vi "Is_TestDataInSpec-1组数据相同规格.vi"(0 "相机量测结果":dbl[](array[numeric]), 1 "量测规格":T1 {"上限" format="%#.4g"; "下限" format="%#.4g"}) -> (3 "在规格内":bool, 4 "相机量测结果 out":dbl[](array[numeric]), 5 "数组":bool[](array[boolean]))   [LabVIEW 2014]
uses:
  Controls/TestThreshold.ctl
panel:
  # "~"
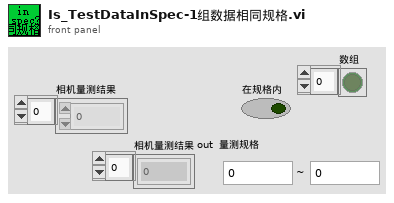
[diagram p1: front panel]
types:
  T1 = typedef "TestThreshold.ctl" = cluster{"下限":dbl, "上限":dbl}
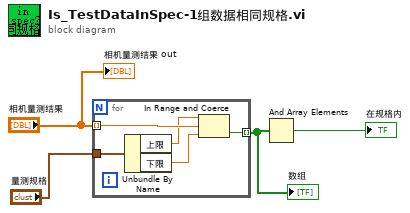
[diagram p0: block diagram]
diagram:
  n1 = for {
    tunnel: "相机量测结果" -> [w9] mode=indexing
    tunnel: [w6] -> w3 mode=indexing
    tunnel: "量测规格" -> [w5]
    n2 = Unbundle By Name(w5) -> ("上限"=w7:dbl, "下限"=w8:dbl)
    n3 = In Range and Coerce(upper limit=w7, x=w9, lower limit=w8) -> (In Range?=w6:bool)  [unwired: 1 out]
  }
  "数组" <- w3
  n4 = And Array Elements(Boolean array=w3) -> (logical AND=→"在规格内":bool)
  "相机量测结果 out" <- "相机量测结果"
